vi "CentralStorage.RequestVarArray.vi"(8 "Error In":errorcluster, 10 "VariantArray":variant[](array[variant]), 11 "CentralStorage (optional)":refnum<data-value>) -> (0 "Error Out":errorcluster, 2 "Output_Ref":refnum<data-value>, 3 "CentralStorage":refnum<data-value>)   [LabVIEW 2016, in "CentralStorage.lvclass"]
uses:
  CentralStorage.lvclass
  CentralStorage.ReferenceRequest.ctl
  CentralStorage.DataTypes.ctl
  CentralStorage.lvclass/CentralStorage.ctl
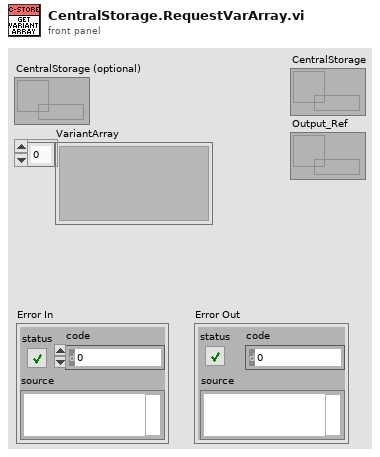
[diagram p1: front panel]
types:
  T1 = typedef "CentralStorage.lvclass/CentralStorage.DataTypes.ctl" = enum16{"Variant Array", "Variant", "Waveform"}
  T2 = typedef "CentralStorage.lvclass/CentralStorage.ReferenceRequest.ctl" = cluster{"Caller":string, "DataType":T1, "Data":variant}
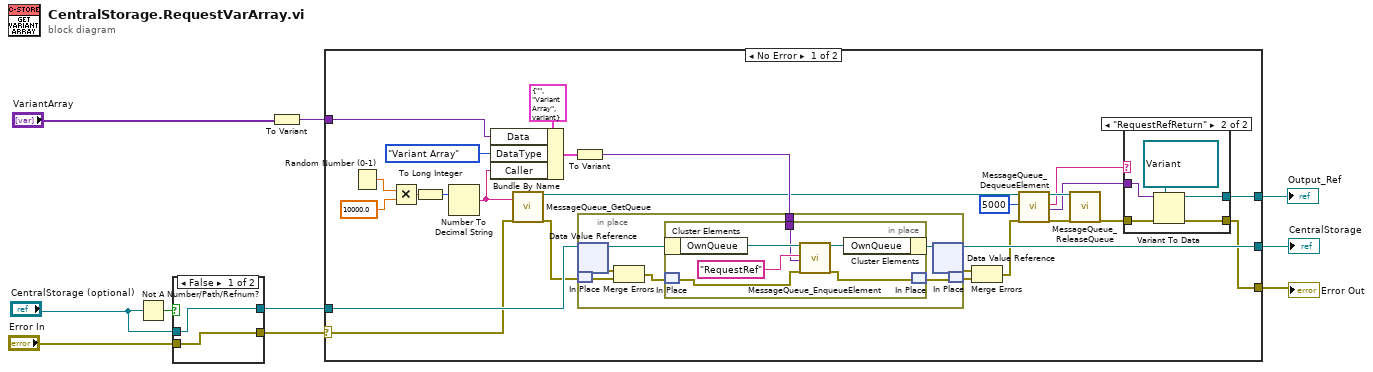
[diagram p0: block diagram]
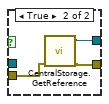
[diagram p4: hidden frame]
diagram:
  n1 = Not A Number/Path/Refnum?(number/path/refnum="CentralStorage (optional)") -> (NaN/Path/Refnum?=w8:bool)
  n2 = case shown="False" w8 {
    tunnel: "CentralStorage (optional)" -> [w12 _]
    tunnel: "Error In" -> [w11 w15]
    tunnel: [w12 w13] -> w5
    tunnel: [w11 w14] -> w9
    frame False {
    }
    frame True {
      n3 = call "CentralStorage.GetReference.vi"("Error in"=w15) -> ("Error out"=w14:errorcluster, "CentralStorage"=w13:refnum<data-value>)  [unwired: 9 in]
    }
  }
  n4 = To Variant(anything="VariantArray") -> (Variant=w3:variant)
  n5 = case shown="No Error" w9 {
    selector: w9 -> [w29 w62]
    tunnel: [w17 w62] -> w10
    tunnel: w5 -> [w41 w61]
    tunnel: [w40 w61] -> w4
    tunnel: w3 -> [w33 _]
    tunnel: [w16 _] -> w1
    frame No Error {
      n6 = Random Number (0-1)() -> (number: 0 to 1=w37:dbl)
      n7 = Multiply(x=w37, y=10000.0) -> (x*y=w38:dbl)
      n8 = To Long Integer(number=w38) -> (32bit integer=w39:i32)
      n9 = Number To Decimal String(number=w39) -> (decimal integer string=w30:string)  [unwired: 1 in]
      n10 = Bundle By Name(cluster=T2 {"Caller"="", "DataType"=enum."Variant Array", "Data"=variant} ("ReferenceRequest"), "Data"=w33, "DataType"=CentralStorage.DataTypes."Variant Array", "Caller"=w30) -> (w27:T2)
      n11 = call "MessageQueue_GetQueue.vi"("Name"=w30, "ErrorIn"=w29) -> ("QueueOut"=w22:refnum<queue>, "ErrorOut"=w28:errorcluster)  [unwired: 15 in, 1 out]
      n12 = To Variant(anything=w27) -> (Variant=w26:variant)
      n13 = in-place {
        in-place-border: w26 -> [w48]
        n14 = in-place-dvr #1(w41) -> (w54:refnum<class "CentralStorage.lvclass">, w52:errorcluster)
        n15 = in-place-match #2(w28) -> (w51:errorcluster)
        n16 = Merge Errors(w52, w51) -> (w50:errorcluster)
        n17 = in-place {
          in-place-border: w48 -> [w55]
          n18 = in-place-cluster #3(w54) -> ("OwnQueue"=w60:refnum<queue>)
          n19 = in-place-match #4(w50) -> (w57:errorcluster)
          n20 = call "MessageQueue_EnqueueElement.vi"("QueueIn"=w60, "Message"="RequestRef", "Data"=w55, "ErrorIn"=w57) -> ("QueueOut"=w59:refnum<queue>, "ErrorOut"=w56:errorcluster)  [unwired: 14 in]
          n21 = in-place-cluster #3("OwnQueue"=w59) -> (w53:refnum<class "CentralStorage.lvclass">)
          n22 = in-place-match #4(w56) -> (w49:errorcluster)
        }
        n23 = in-place-dvr #1(w53) -> (w40:refnum<data-value>, w31:errorcluster)
        n24 = in-place-match #2(w49) -> (w32:errorcluster)
      }
      n25 = Merge Errors(w31, w32) -> (w25:errorcluster)
      n26 = call "MessageQueue_DequeueElement.vi"("QueueIn"=w22, "Timeout"=5000, "ErrorIn"=w25) -> ("QueueOut"=w23:refnum<queue>, "Message"=w20:string, "Data"=w19:variant, "ErrorOut"=w24:errorcluster)  [unwired: 12 in, 1 out]
      n27 = call "MessageQueue_ReleaseQueue.vi"("QueueIn"=w23, "ErrorIn"=w24) -> ("ErrorOut"=w18:errorcluster)  [unwired: 15 in, 2 out]
      n28 = case shown="\"RequestRefReturn\"" w20 {
        tunnel: w19 -> [_ w45]
        tunnel: w18 -> [w42 w47]
        tunnel: [w42 w46] -> w17
        tunnel: [_ w43] -> w16
        frame Default {
        }
        frame "RequestRefReturn" {
          n29 = Variant To Data(error in=w47, type=refnum<data-value> refnum ("Output_Ref 2"), Variant=w45) -> (data=w43:refnum<data-value>, error out=w46:errorcluster)
        }
      }
    }
    frame Error {
    }
  }
  "Error Out" <- w10
  "CentralStorage" <- w4
  "Output_Ref" <- w1
